vi "ReadSignals.Compile.vi"(8 "error in (no error)":errorcluster, 10 "Settings":T4[](array[typedef]) {"Signal.Cmd.Refs"."Signal Refs" format="%.0x"; "Signal.Cmd.Info"."Signals"."Byte Order" items=["Little Endian", "Big Endian"]; "Signal.Cmd.Info"."Signals"."Data Type" items=["Signed", "Unsigned", "IEEE Float"]; "Settings.Refs"."Signal Refs" format="%.0x"; "Signal.Resp.Refs"."Signal Refs" format="%.0x"; "Signal.Resp.Info"."Signals"."Byte Order" items=["Little Endian", "Big Endian"]; "Signal.Resp.Info"."Signals"."Data Type" items=["Signed", "Unsigned", "IEEE Float"]; "Trigger.Refs"."Signal Refs" format="%.0x"; "Status.Refs"."Signal Refs" format="%.0x"}, 11 "Lookups in":variant) -> (0 "error out":errorcluster, 1 "Signal Info":T1[](array[typedef]) {"Signals"."Byte Order" items=["Little Endian", "Big Endian"]; "Signals"."Data Type" items=["Signed", "Unsigned", "IEEE Float"]}, 2 "Refs":T7 {"VS Refs" format="%.0x"}, 3 "Lookups":variant)   [LabVIEW 2019, in "Diagnostics Addon System Explorer.lvlib"]
uses:
  Diagnostics Addon System Explorer.lvlib
  <vilib>/NI VeriStand/Custom Device API/Custom Device Item Ref.ctl
  Types/Service.Export.ctl
  Types/Frame.Ref.ctl
  Addon Shared/Types/Type.ctl
  Addon Shared/Types/Frame.Compile.ctl
  Addon Shared/Types/Signal.ctl
  Addon Shared/Types/Frame.Lookup.Info.ctl
  Addon Shared/SubVIs/Constants.vi
  Addon Shared/Diagnostics Addon Shared.lvlib
  <vilib>/NI VeriStand/Custom Device API/Custom Device API.lvlib
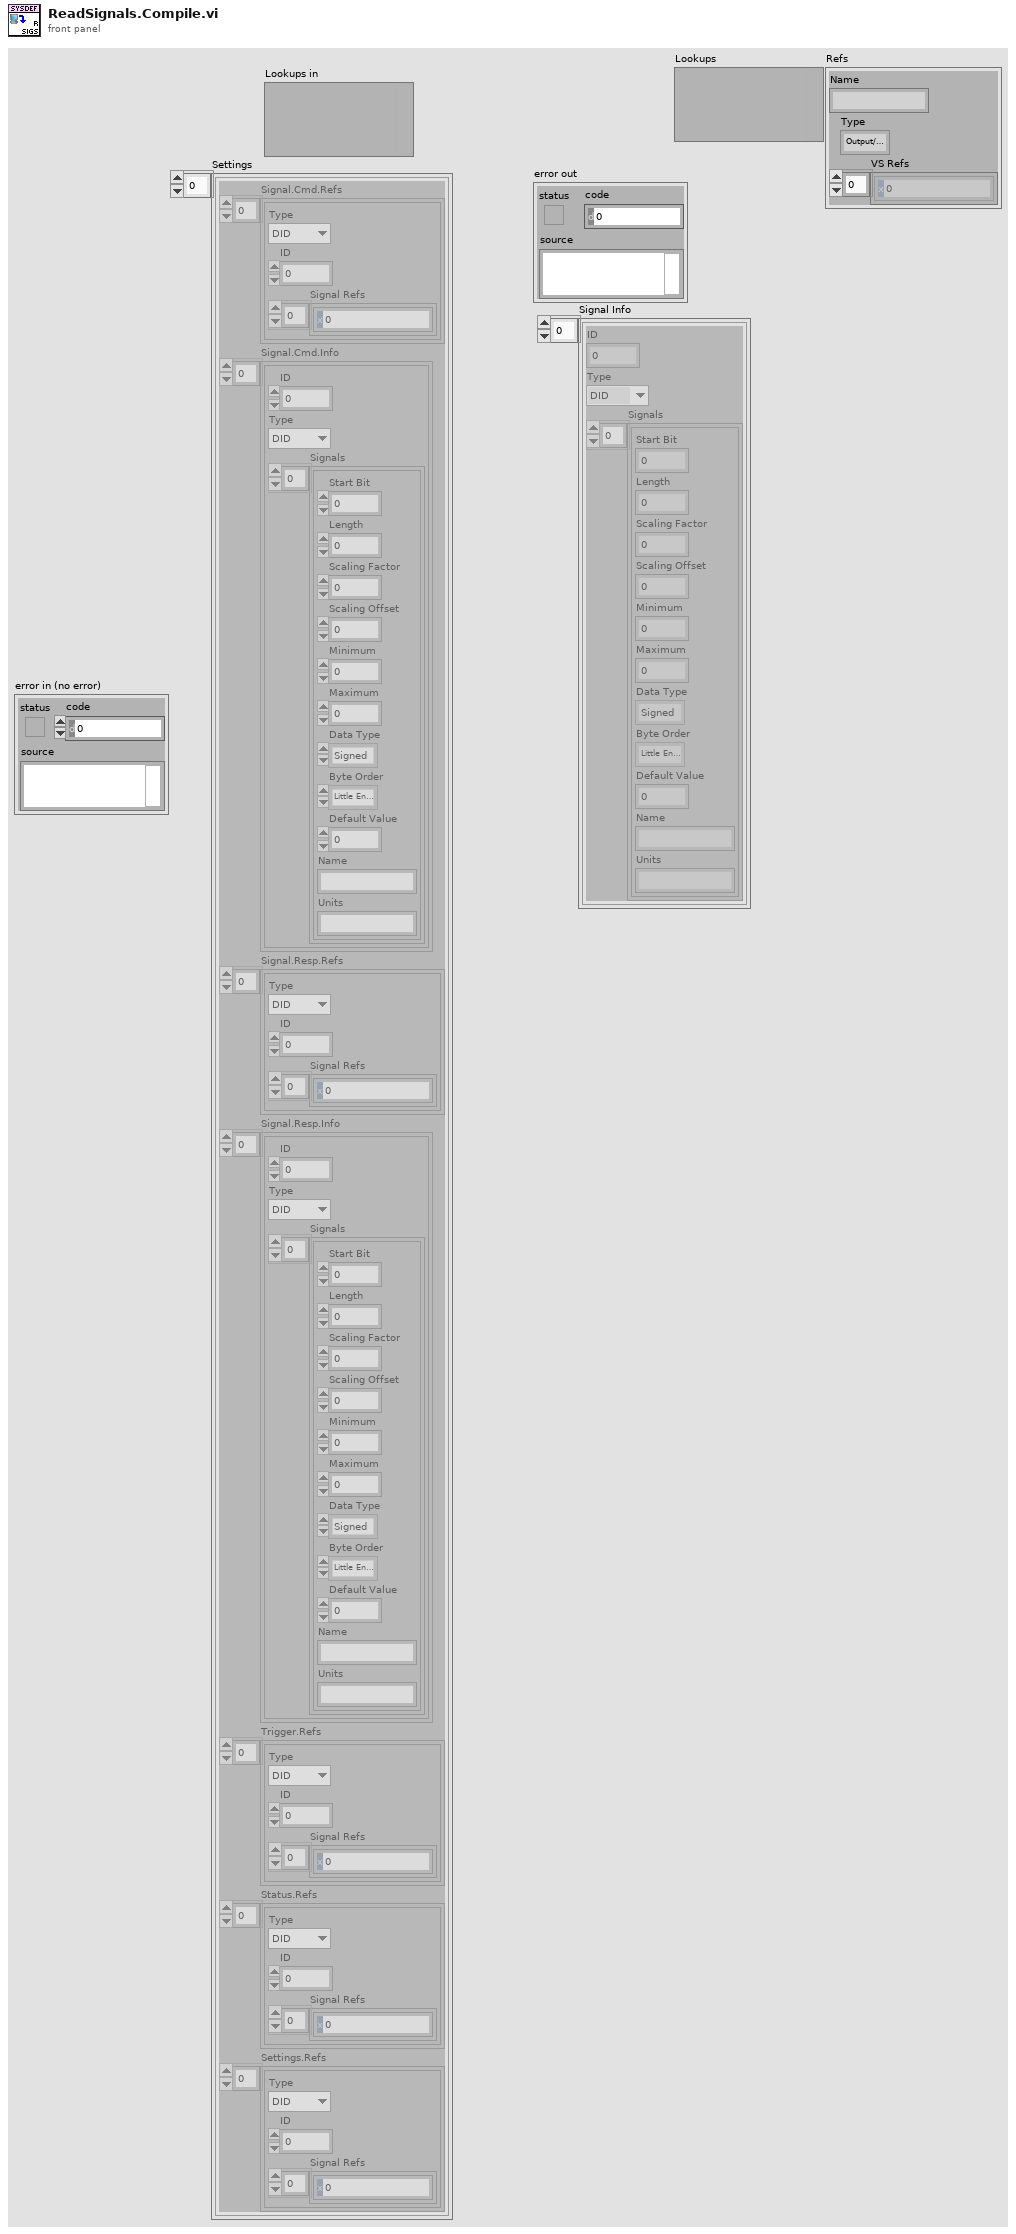
[diagram p1: front panel]
types:
  T1 = typedef "Diagnostics Addon Shared.lvlib/Frame.Compile.ctl" = cluster{"ID":u32, "Type":T2, "Signals":T3[]}
  T2 = typedef "Diagnostics Addon Shared.lvlib/Type.ctl" = enum16{"DID", "CDID", "PID", "CPID", "Read Memory", "Write Memory", "IO Control", "Routine Start", "Routine Request", "Routine Stop", "User Defined", "DTC Control", "Clear DTCs", "Read DTCs", "Start DTCs", "DTC Change Count", "Tester Present", "Unlock ECU", "Reset ECU", "Diag Session Control", "Communication Control", "DPID Control", "Poll Control", "Diag CAN Control"}
  T3 = typedef "Diagnostics Addon Shared.lvlib/Signal.ctl" = cluster{"Start Bit":u32, "Length":u32, "Scaling Factor":dbl, "Scaling Offset":dbl, "Minimum":dbl, "Maximum":dbl, "Data Type":u32, "Byte Order":u32, "Default Value":dbl, "Name":string, "Units":string}
  T4 = typedef "Diagnostics Addon System Explorer.lvlib/Service.Export.ctl" = cluster{"Signal.Cmd.Refs":T5[], "Signal.Cmd.Info":T1[], "Signal.Resp.Refs":T5[], "Signal.Resp.Info":T1[], "Trigger.Refs":T5[], "Status.Refs":T5[], "Settings.Refs":T5[]}
  T5 = typedef "Diagnostics Addon System Explorer.lvlib/Frame.Ref.ctl" = cluster{"Type":T2, "ID":u32, "Signal Refs":T6[]}
  T6 = typedef "Custom Device API.lvlib/Custom Device Item Ref.ctl" = u64
  T7 = cluster{"Name":string, "Type":enum16{"Output/Write", "Input/Read", "Input/ReadWrite"}, "VS Refs":T6[]}
  T8 = enum16{"Output/Write", "Input/Read", "Input/ReadWrite"}
  T9 = typedef "Diagnostics Addon Shared.lvlib/Frame.Lookup.Info.ctl" = cluster{"Offset":i32, "Length":i32, "ByteLength":u16}
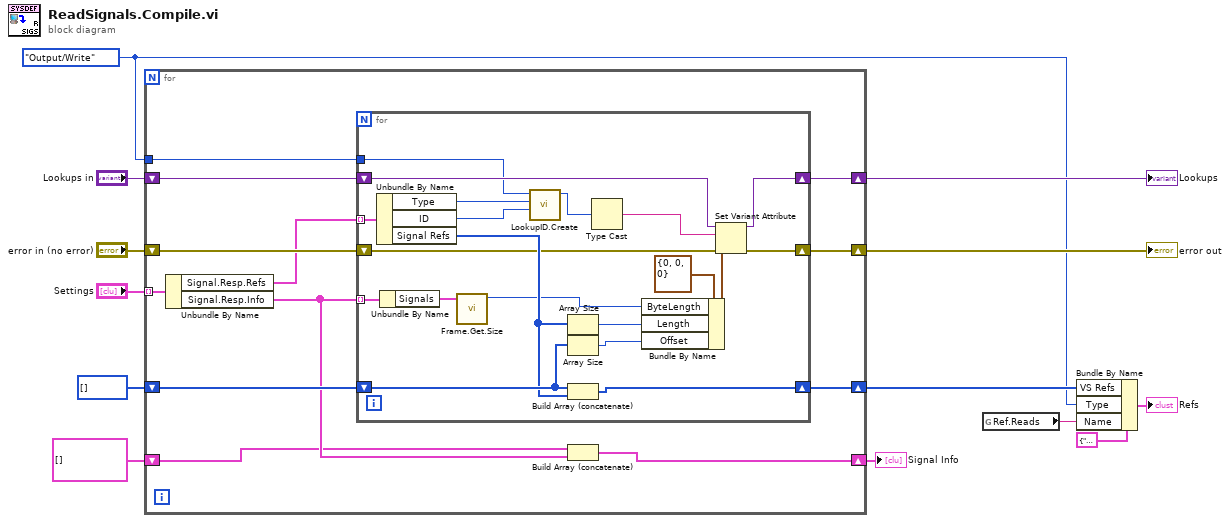
[diagram p0: block diagram]
diagram:
  w1 = T8."Output/Write" ("Type")
  n1 = for {
    shift-right: [w20] -> w5
    shift-left: "error in (no error)" -> [w25]
    shift-right: [w23] -> w11
    shift-left: "Lookups in" -> [w22]
    tunnel: "Settings" -> [w19] mode=indexing
    shift-right: [w21] -> w7
    shift-left: T6[] [] ("Signal Refs") -> [w24]
    shift-right: [w15] -> w3
    shift-left: T1[] [] -> [w16]
    tunnel: w1 -> [w14]
    n2 = Unbundle By Name(w19) -> ("Signal.Resp.Refs"=w18:T5[], "Signal.Resp.Info"=w17:T1[])
    n3 = for {
      tunnel: w18 -> [w35] mode=indexing
      shift-right: [w44] -> w21
      shift-left: w24 -> [w45]
      shift-right: [w36] -> w23
      shift-left: w22 -> [w40]
      shift-right: [w38] -> w20
      shift-left: w25 -> [w33]
      tunnel: w17 -> [w32] mode=indexing
      tunnel: w14 -> [w26]
      n4 = Unbundle By Name(w35) -> ("Type"=w27:T2, "ID"=w29:u32, "Signal Refs"=w34:T6[])
      n5 = Unbundle By Name(w32) -> ("Signals"=w31:T3[])
      n6 = call "Frame.Get.Size.vi"("Parameters"=w31) -> ("Bytes"=w30:u32)  [unwired: 10 in]
      n7 = call "LookupID.Create.vi"("Serivce ID"=w29, "Service Type"=w27, "Direction"=w26) -> ("Result"=w28:u64)  [unwired: 8 in]
      n8 = Array Size(array=w34) -> (size(s)=w43:i32)
      n9 = Array Size(array=w45) -> (size(s)=w39:i32)
      n10 = Build Array (concatenate)(w45, w34) -> (w44:T6[])
      n11 = Type Cast(x=w28) -> (*(type *) &x=w37:string)  [unwired: 1 in]
      n12 = Bundle By Name(cluster=T9 {"Offset"=0, "Length"=0, "ByteLength"=0}, "ByteLength"=w30, "Length"=w43, "Offset"=w39) -> (w41:T9)
      n13 = Set Variant Attribute(Variant=w40, name=w37, value=w41, error in=w33) -> (Variant out=w36:variant, error out=w38:errorcluster)  [unwired: 1 out]
    }
    n14 = Build Array (concatenate)(w16, w17) -> (w15:T1[])
  }
  "error out" <- w5
  "Lookups" <- w11
  "Signal Info" <- w3
  n15 = global read "Constants.vi" "Ref.Reads"() -> (w8:string)
  n16 = Bundle By Name(cluster=T7 {"Name"="", "Type"=enum."Output/Write", "VS Refs"=[]} ("Group"), "VS Refs"=w7, "Type"=w1, "Name"=w8) -> (→"Refs":T7)
